vi "StartLogFile.vi"(0 "Path In":path, 1 "Line 1":string, 2 "Line 2":string, 3 "Line 3":string, 4 "Line 4":string, 5 "Line 5":string, 6 "Log File Header":string, 8 "Extension":string, 10 "UTC format":bool, 13 "error in (no error)":errorcluster) -> (14 "Path":path, 19 "error out":errorcluster)   [LabVIEW 2013]
doc: "Starts a log file, taking a path and header name. The header name will be run thorugh Date/Time Formatting, so it can contain entries such as %y%m%d. The default extension is currently *.tsv, and cannot be modified. This is the best extension to use in general, especially since in some locales, comma (i.e. *.csv) is used for the decimal place."
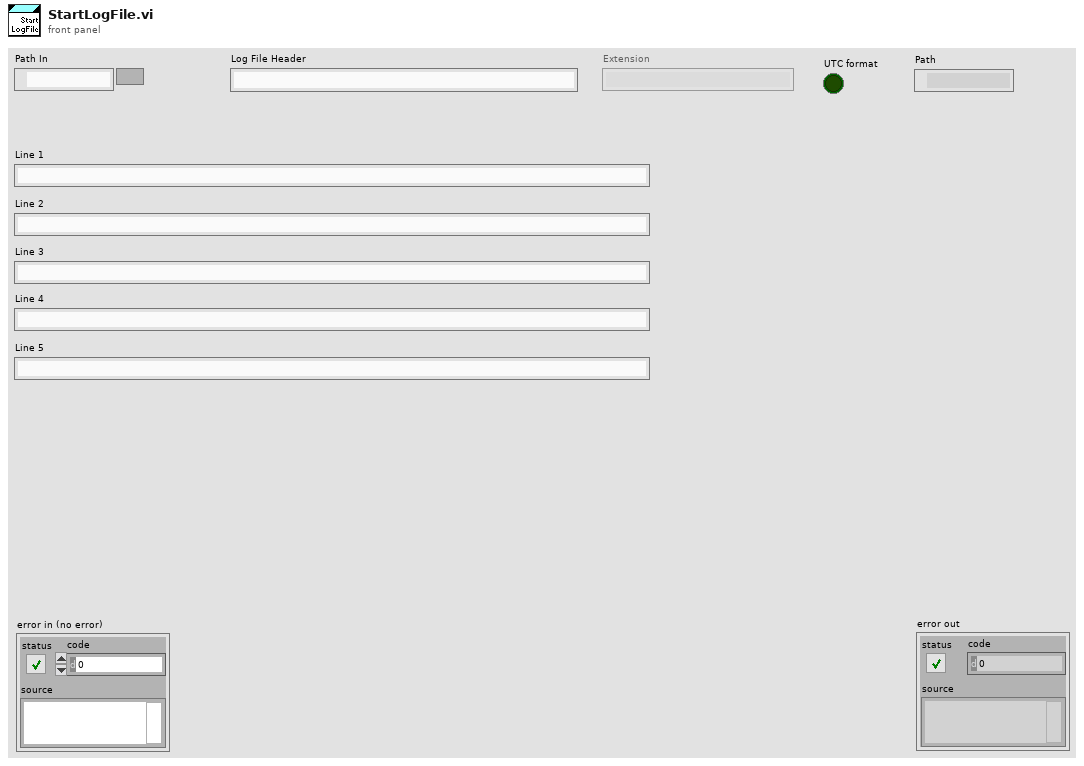
[diagram p1: front panel]
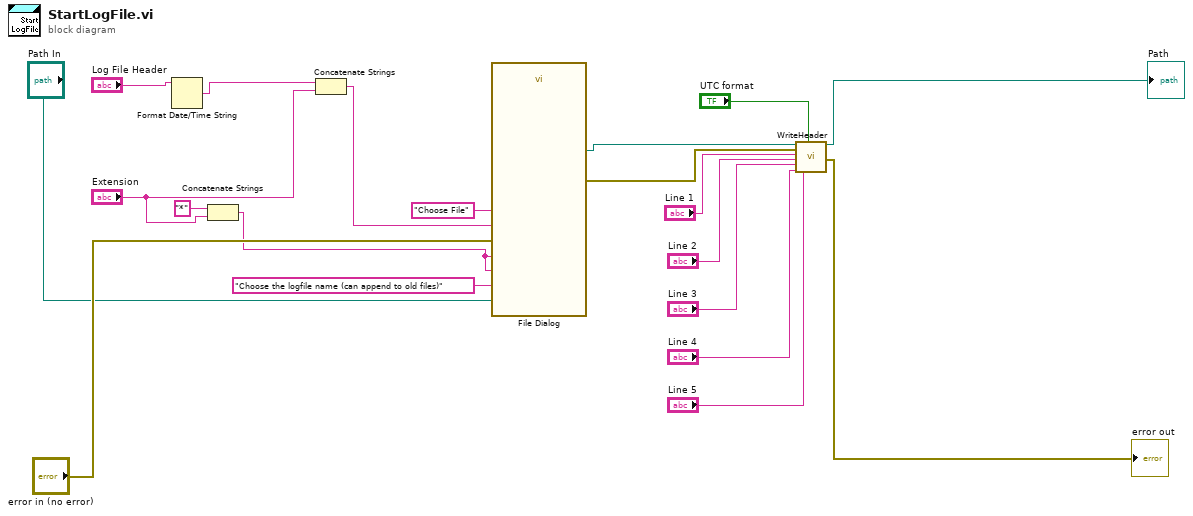
[diagram p0: block diagram]
diagram:
  n1 = Format Date/Time String(time format string (%c)="Log File Header") -> (date/time string=w12:string)  [unwired: 2 in]
  n2 = Concatenate Strings("*" ("string"), "Extension") -> (w14:string)
  n3 = Concatenate Strings(w12, "Extension") -> (w17:string)
  n4 = call "File Dialog"("start path"="Path In", "prompt"="Choose the logfile name (can append to old files)", "button label"="Choose File", "default name"=w17, "error in"="error in (no error)", "pattern (all files)"=w14, "pattern label"=w14) -> ("selected path"=w10:path, "error out"=w2:errorcluster)  [unwired: 5 in, 2 out]
  n5 = call "WriteHeader.vi"("Path In"=w10, "error in (no error)"=w2, "Line 1"="Line 1", "Line 2"="Line 2", "Line 3"="Line 3", "Line 4"="Line 4", "Line 5"="Line 5", "UTC format"="UTC format") -> ("Path"=→"Path":path, "error out"=→"error out":errorcluster)  [unwired: 10 in]
